vi "range_between_example.vi"() -> ()   [LabVIEW 2018]
panel:
  out "Boolean 2":bool
  out "Ambos":bool
  out "In Range?":bool
  in  "x":dbl
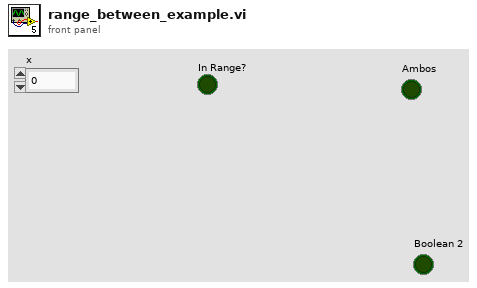
[diagram p1: front panel]
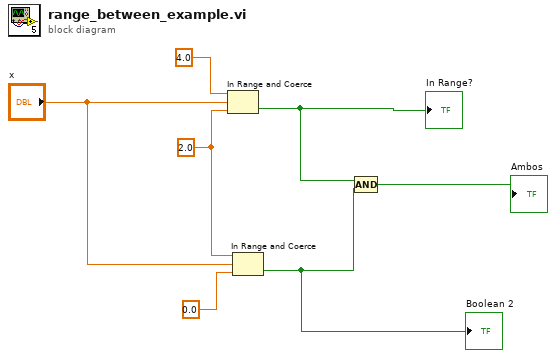
[diagram p0: block diagram]
diagram:
  w5 = 2.0 ("lower limit")
  n1 = In Range and Coerce(upper limit=4.0, x="x", lower limit=w5) -> (In Range?=w3:bool)  [unwired: 1 out]
  "In Range?" <- w3
  n2 = In Range and Coerce(upper limit=w5, x="x", lower limit=0.0) -> (In Range?=w1:bool)  [unwired: 1 out]
  "Boolean 2" <- w1
  n3 = Compound Arithmetic op=AND(w3, w1) -> (→"Ambos":bool)
